vi "FAIR_GROUNDS_TEST_basaeline.vi"(1 "FIRE":bool, 2 "REVERSE":bool, 3 "Intake Motor":bool, 4 "OVERRIDE":bool, 5 "OVERRIDE 2":bool, 8 "BB1":bool, 9 "1":bool, 10 "BB2":bool, 11 "2":bool, 12 "BB3":bool, 13 "3":bool, 14 "BB4":bool) -> (20 "Ball Count":dbl, 21 "Intake motor":dbl, 22 "Motor A 2":dbl, 23 "Motor B 3":dbl, 24 "Motor C":dbl)   [LabVIEW 2011]
panel:
  in  "Prime":dbl(knob)=0.20200759564815568 scale=0.0..1.0
  in  "FIRE":dbl(knob)=0.5049245430258039 scale=0.0..1.0
  out "C from 3":bool
  out "B from 2":bool
  out "A from 1":bool
  out "BSB State":enum16{"Ball Entered"}(ring)
  out "BSC":bool
  out "BSB":bool
  out "BSA":bool
  out "MC":enum16{"Stopped", "Foward", "Reverse"}(ring)
  out "MA":enum16{"Stopped", "Foward", "Reverse"}(ring)
  out "MB":enum16{"Stopped", "Foward", "Reverse"}(ring)
  out "Intake motor":bool
  out "C Status":string
  out "B Status":string
  out "A Status":string
  out "Ball System State":string
  out "Primed":bool
  out "MA":bool
  out "MB":bool
  out "MC":bool
  # "Upper System"
  # "Upper/Middle System (U/M)"
  # "Ball systems"
  # "Vacant = Black (T)\nOccupied = Orange (F)"
  # "Lower/Middle System (L/M)"
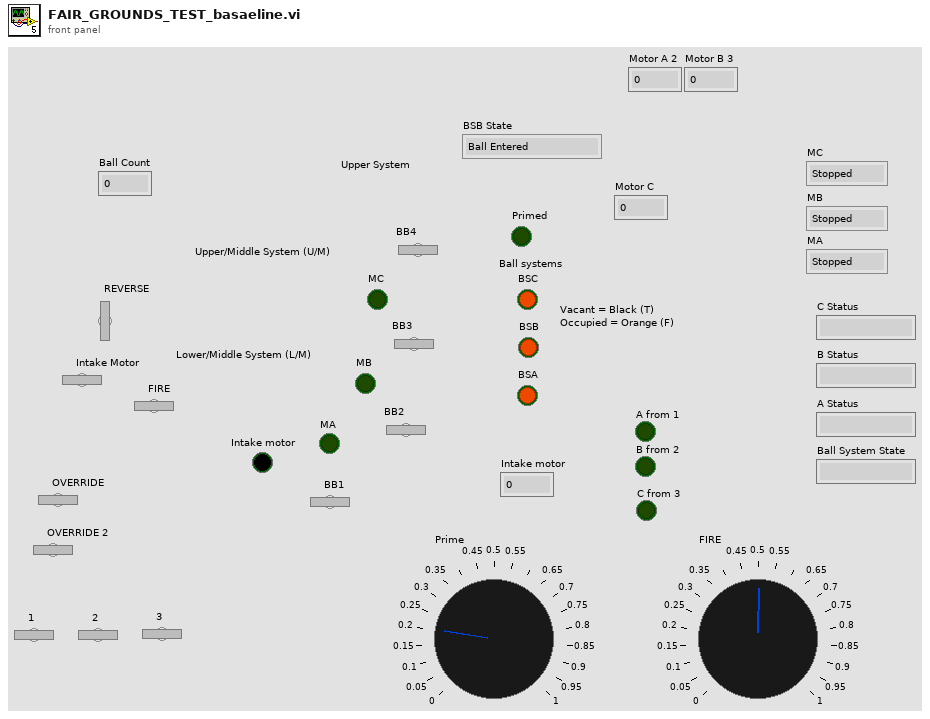
[diagram p1: front panel]
types:
  T1 = enum16{"Ball Entered", "Ball Stopped", "Ball Moveing", "Ball Leaving"}
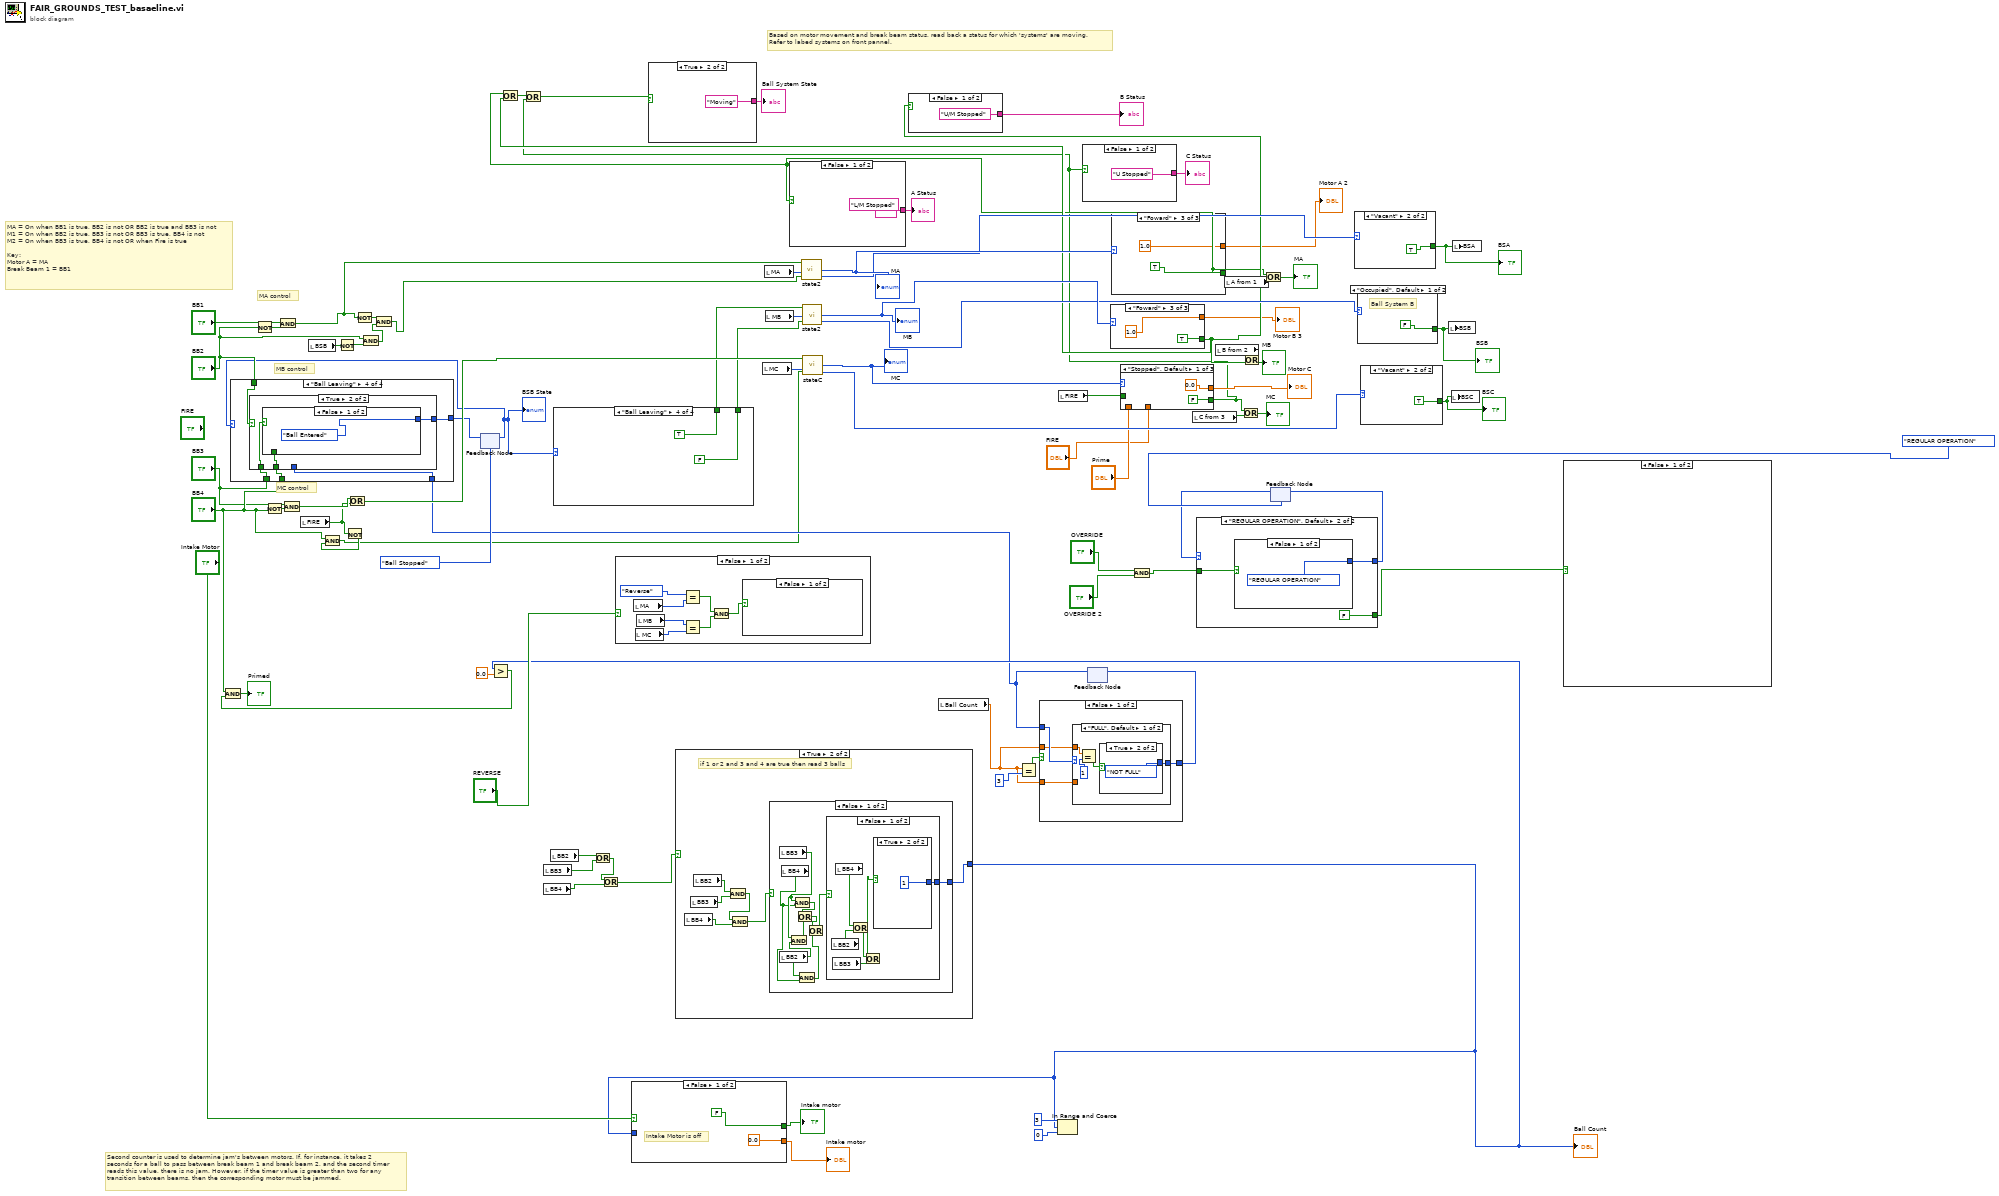
[diagram p0: block diagram]
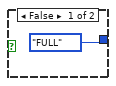
[diagram p2: hidden frame]
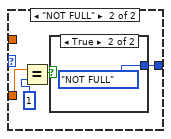
[diagram p3: hidden frame]
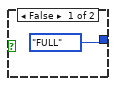
[diagram p4: hidden frame]
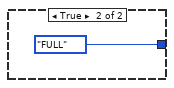
[diagram p5: hidden frame]
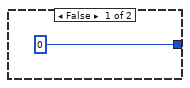
[diagram p6: hidden frame]
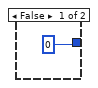
[diagram p7: hidden frame]
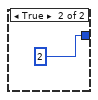
[diagram p8: hidden frame]
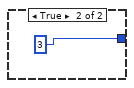
[diagram p9: hidden frame]
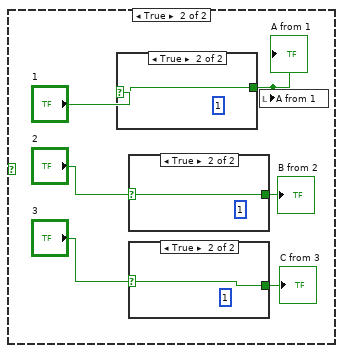
[diagram p10: hidden frame]
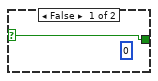
[diagram p11: hidden frame]
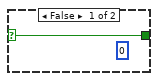
[diagram p12: hidden frame]
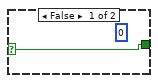
[diagram p13: hidden frame]
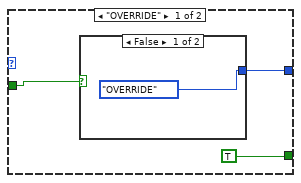
[diagram p14: hidden frame]
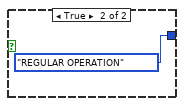
[diagram p15: hidden frame]
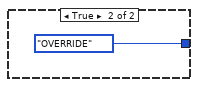
[diagram p16: hidden frame]
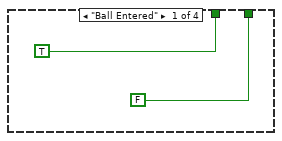
[diagram p17: hidden frame]
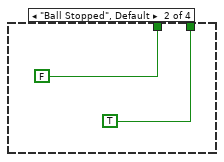
[diagram p18: hidden frame]
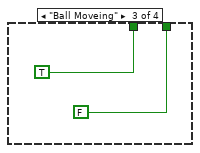
[diagram p19: hidden frame]
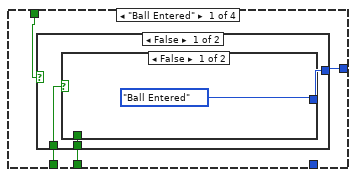
[diagram p20: hidden frame]
diagram:
  # "MC control"
  # "MB control"
  # "MA control"
  # "Second counter is used to determine jam's between motors. If, for instance, it takes 2\nseconds for a ball to pass between break beam 1 and break beam 2, and the second timer\nreads this value, there is no jam. However, if the timer value is greater than two for any\ntransition between beams, then the corresponding motor must be jammed."
  # "Based on motor movement and break beam status, read back a status for which 'systems' are moving.\nRefer to labed systems on front pannel."
  # "MA = On when BB1 is true, BB2 is not OR BB2 is true and BB3 is not\nM1 = On when BB2 is true, BB3 is not OR BB3 is true, BB4 is not\nM2 = On when BB3 is true, BB4 is not OR when Fire is true\n\nKey:\nMotor A = MA\nBreak Beam 1 = BB1"
  n1 = Not(x="BB2") -> (.not. x?=w59:bool)
  n2 = Not(x="BB4") -> (.not. x?=w58:bool)
  n3 = And(x="BB1", y=w59) -> (x .and. y?=w46:bool)
  n4 = And(x="BB3", y=w58) -> (x .and. y?=w57:bool)
  n5 = local read "FIRE"() -> (w16:bool)
  n6 = local read "BSB"() -> (w56:bool)
  n7 = Not(x=w56) -> (.not. x?=w55:bool)
  n8 = Not(x=w16) -> (.not. x?=w4:bool)
  n9 = And(x="BB4", y=w4) -> (x .and. y?=w3:bool)
  n10 = Or(x=w57, y=w16) -> (x .or. y?=w47:bool)
  n11 = Not(x=w46) -> (.not. x?=w52:bool)
  n12 = And(x="BB2", y=w55) -> (x .and. y?=w54:bool)
  n13 = And(x=w52, y=w54) -> (x .and. y?=w53:bool)
  n14 = feedback #1(T1."Ball Stopped") -> (w37:T1)
  "BSB State" <- w37
  n15 = local read "BB4"() -> (w19:bool)
  n16 = local read "BB3"() -> (w18:bool)
  n17 = local read "BB2"() -> (w20:bool)
  n18 = case shown="\"Ball Leaving\"" w37 {
    tunnel: [TRUE FALSE TRUE TRUE] -> w40
    tunnel: [FALSE TRUE FALSE FALSE] -> w39
    frame "Ball Entered" {
    }
    frame "Ball Stopped", Default {
    }
    frame "Ball Moveing" {
    }
    frame "Ball Leaving" {
    }
  }
  n19 = Or(x=w20, y=w18) -> (x .or. y?=w21:bool)
  n20 = Or(x=w21, y=w19) -> (x .or. y?=w17:bool)
  n21 = case shown="False" "REVERSE" {
    frame False {
      n22 = local read "MA"() -> (w96:enum16{"Stopped", "Foward", "Reverse"})
      n23 = local read "MC"() -> (w94:enum16{"Stopped", "Foward", "Reverse"})
      n24 = local read "MB"() -> (w95:enum16{"Stopped", "Foward", "Reverse"})
      n25 = Equal?(x=enum16{"Stopped", "Foward", "Reverse"}."Reverse" ("value"), y=w96) -> (x = y?=w92:bool)
      n26 = Equal?(x=w95, y=w94) -> (x = y?=w93:bool)
      n27 = And(x=w92, y=w93) -> (x .and. y?=w91:bool)
      n28 = case shown="False" w91 {
        frame False {
        }
        frame True {
          w98 = enum16{"Stopped", "Foward", "Reverse"}."Stopped" ("value")
          n29 = local write "MA"(w98) -> ()
          n30 = local write "MB"(w98) -> ()
          n31 = local write "MC"(w98) -> ()
        }
      }
    }
    frame True {
      w99 = enum16{"Stopped", "Foward", "Reverse"}."Reverse" ("MB")
      n32 = local write "MC"(w99) -> ()
      n33 = local write "MA"(w99) -> ()
      n34 = local write "MB"(w99) -> ()
    }
  }
  n35 = case shown="True" w17 {
    tunnel: [0 w102] -> w15
    frame False {
    }
    frame True {
      # "if 1 or 2 and 3 and 4 are true then read 3 balls"
      n36 = local read "BB4"() -> (w103:bool)
      n37 = local read "BB3"() -> (w104:bool)
      n38 = local read "BB2"() -> (w105:bool)
      n39 = And(x=w105, y=w104) -> (x .and. y?=w106:bool)
      n40 = And(x=w106, y=w103) -> (x .and. y?=w101:bool)
      n41 = case shown="False" w101 {
        tunnel: [w115 3] -> w102
        frame False {
          n42 = local read "BB3"() -> (w112:bool)
          n43 = local read "BB2"() -> (w111:bool)
          n44 = local read "BB4"() -> (w110:bool)
          n45 = And(x=w112, y=w111) -> (x .and. y?=w113:bool)
          n46 = And(x=w112, y=w110) -> (x .and. y?=w114:bool)
          n47 = Or(x=w114, y=w113) -> (x .or. y?=w109:bool)
          n48 = And(x=w111, y=w110) -> (x .and. y?=w107:bool)
          n49 = Or(x=w109, y=w107) -> (x .or. y?=w108:bool)
          n50 = case shown="False" w108 {
            tunnel: [w121 2] -> w115
            frame False {
              n51 = local read "BB2"() -> (w120:bool)
              n52 = local read "BB3"() -> (w118:bool)
              n53 = local read "BB4"() -> (w116:bool)
              n54 = Or(x=w116, y=w120) -> (x .or. y?=w119:bool)
              n55 = Or(x=w119, y=w118) -> (x .or. y?=w117:bool)
              n56 = case shown="True" w117 {
                tunnel: [0 1] -> w121
                frame False {
                }
                frame True {
                }
              }
            }
            frame True {
            }
          }
        }
        frame True {
        }
      }
    }
  }
  "Ball Count" <- w15
  n57 = Greater?(x=w15, y=0.0 ("f")) -> (0:w74:bool)
  n58 = And(x="BB4", y=w74) -> (x .and. y?=→"Primed":bool)
  n59 = case shown="False" "Intake Motor" {
    tunnel: [FALSE w130] -> w77
    tunnel: [0.0 w129] -> w50
    tunnel: w15 -> [_ w128]
    frame False {
      # "Intake Motor is off"
    }
    frame True {
      # "Only allow the intake\nmotor to be on if\nthere are less than\n3 Ballz"
      n60 = Less?(x=w128, y=3) -> (x < y?=w131:bool)
      n61 = case shown="False" w131 {
        selector: w131 -> [_ w136]
        tunnel: [TRUE w136] -> w130
        tunnel: [-1 1] -> w129
        frame False {
        }
        frame True {
        }
      }
    }
  }
  "Intake motor" <- w77
  "Intake motor" <- w50
  n62 = local read "MC"() -> (w70:enum16{"Stopped", "Foward", "Reverse"})
  n63 = local read "MA"() -> (w71:enum16{"Stopped", "Foward", "Reverse"})
  n64 = local read "MB"() -> (w72:enum16{"Stopped", "Foward", "Reverse"})
  n65 = call "state2.vi"("Stop/Transfer"=w53, "State"=w71, "Start"=w46) -> ("Ball State"=w63:enum16{"Occupied", "Vacant"}, "OutState"=w69:enum16{"Stopped", "Foward", "Reverse"})  [unwired: 1 in]
  "MA" <- w69
  n66 = call "state2.vi"("Stop/Transfer"=w39, "State"=w72, "Start"=w40) -> ("Ball State"=w64:enum16{"Occupied", "Vacant"}, "OutState"=w68:enum16{"Stopped", "Foward", "Reverse"})  [unwired: 1 in]
  "MB" <- w68
  n67 = call "stateC.vi"("Stop/Transfer"=w3, "State"=w70, "Start"=w47) -> ("Ball State"=w65:enum16{"Occupied", "Vacant"}, "OutState"=w67:enum16{"Stopped", "Foward", "Reverse"})  [unwired: 1 in]
  "MC" <- w67
  n68 = local read "Ball Count"() -> (w10:dbl)
  n69 = Equal?(x=w10, y=3) -> (x = y?=w13:bool)
  n70 = In Range and Coerce(upper limit=3, x=w15, lower limit=0) -> ()  [unwired: 2 out]
  n71 = local read "FIRE"() -> (w8:bool)
  n72 = feedback #2() -> (w11:enum16{"FULL", "NOT FULL"})  [unwired: 1 in]
  n73 = case shown="\"Ball Leaving\"" w37 {
    tunnel: "BB2" -> [w140 w160 w180 w203]
    tunnel: "BB3" -> [w139 w159 w179 w205]
    tunnel: "BB4" -> [w138 w158 w178 w204]
    tunnel: [w137 w157 w181 w206] -> w38
    tunnel: w11 -> [_ _ w177 w202]
    frame "Ball Entered" {
      n74 = case shown="False" w140 {
        tunnel: [w143 w151] -> w137
        tunnel: w139 -> [w142 w149]
        tunnel: w138 -> [w141 w150]
        frame False {
          n75 = case shown="False" w142 {
            tunnel: [T1."Ball Entered" w146] -> w143
            tunnel: w141 -> [_ w145]
            frame False {
            }
            frame True {
              n76 = case shown="False" w145 {
                tunnel: [T1."Ball Leaving" T1."Ball Stopped"] -> w146
                frame False {
                }
                frame True {
                }
              }
            }
          }
        }
        frame True {
          n77 = case shown="False" w149 {
            tunnel: [T1."Ball Entered" w154] -> w151
            tunnel: w150 -> [_ w153]
            frame False {
            }
            frame True {
              n78 = case shown="False" w153 {
                tunnel: [T1."Ball Leaving" T1."Ball Stopped"] -> w154
                frame False {
                }
                frame True {
                }
              }
            }
          }
        }
      }
    }
    frame "Ball Stopped", Default {
      n79 = case shown="True" w160 {
        tunnel: [w163 w171] -> w157
        tunnel: w159 -> [w162 w169]
        tunnel: w158 -> [w161 w170]
        frame False {
          n80 = case shown="False" w162 {
            tunnel: [T1."Ball Stopped" w166] -> w163
            tunnel: w161 -> [_ w165]
            frame False {
            }
            frame True {
              n81 = case shown="True" w165 {
                tunnel: [T1."Ball Leaving" T1."Ball Stopped"] -> w166
                frame False {
                }
                frame True {
                }
              }
            }
          }
        }
        frame True {
          n82 = case shown="False" w169 {
            tunnel: [T1."Ball Entered" w174] -> w171
            tunnel: w170 -> [_ w173]
            frame False {
            }
            frame True {
              n83 = case shown="True" w173 {
                tunnel: [T1."Ball Leaving" T1."Ball Stopped"] -> w174
                frame False {
                }
                frame True {
                }
              }
            }
          }
        }
      }
    }
    frame "Ball Moveing" {
      n84 = case shown="False" w180 {
        tunnel: [w185 w196] -> w181
        tunnel: w179 -> [w184 w194]
        tunnel: w178 -> [w183 w195]
        tunnel: w177 -> [w182 _]
        frame False {
          n85 = case shown="False" w184 {
            tunnel: [w187 w191] -> w185
            tunnel: w183 -> [_ w190]
            tunnel: w182 -> [w186 _]
            frame False {
              n86 = case shown="\"NOT FULL\"" w186 {
                tunnel: [T1."Ball Moveing" T1."Ball Stopped"] -> w187
                frame "FULL", Default {
                }
                frame "NOT FULL" {
                }
              }
            }
            frame True {
              n87 = case shown="True" w190 {
                tunnel: [T1."Ball Moveing" T1."Ball Stopped"] -> w191
                frame False {
                }
                frame True {
                }
              }
            }
          }
        }
        frame True {
          n88 = case shown="False" w194 {
            tunnel: [T1."Ball Entered" w199] -> w196
            tunnel: w195 -> [_ w198]
            frame False {
            }
            frame True {
              n89 = case shown="False" w198 {
                tunnel: [T1."Ball Leaving" T1."Ball Stopped"] -> w199
                frame False {
                }
                frame True {
                }
              }
            }
          }
        }
      }
    }
    frame "Ball Leaving" {
      n90 = case shown="True" w203 {
        tunnel: [w210 w221] -> w206
        tunnel: w205 -> [w209 w219]
        tunnel: w204 -> [w208 w220]
        tunnel: w202 -> [w207 _]
        frame False {
          n91 = case shown="False" w209 {
            tunnel: [w212 w216] -> w210
            tunnel: w208 -> [_ w215]
            tunnel: w207 -> [w211 _]
            frame False {
              n92 = case shown="\"NOT FULL\"" w211 {
                tunnel: [T1."Ball Moveing" T1."Ball Stopped"] -> w212
                frame "FULL", Default {
                }
                frame "NOT FULL" {
                }
              }
            }
            frame True {
              n93 = case shown="True" w215 {
                tunnel: [T1."Ball Leaving" T1."Ball Stopped"] -> w216
                frame False {
                }
                frame True {
                }
              }
            }
          }
        }
        frame True {
          n94 = case shown="False" w219 {
            tunnel: [T1."Ball Entered" w224] -> w221
            tunnel: w220 -> [_ w223]
            frame False {
            }
            frame True {
              n95 = case shown="False" w223 {
                tunnel: [T1."Ball Leaving" T1."Ball Stopped"] -> w224
                frame False {
                }
                frame True {
                }
              }
            }
          }
        }
      }
    }
  }
  n96 = feedback-in #1(w38) -> ()
  n97 = case shown="False" w13 {
    tunnel: w11 -> [w230 _]
    tunnel: [w229 enum16{"FULL", "NOT FULL"}."FULL"] -> w12
    tunnel: w10 -> [w228 _]
    tunnel: w10 -> [w227 _]
    frame False {
      n98 = case shown="\"FULL\", Default" w230 {
        tunnel: [w231 w240] -> w229
        tunnel: w228 -> [_ w239]
        tunnel: w227 -> [w232 _]
        frame "FULL", Default {
          n99 = Equal?(x=w232, y=1) -> (x = y?=w234:bool)
          n100 = case shown="True" w234 {
            tunnel: [enum16{"FULL", "NOT FULL"}."FULL" enum16{"FULL", "NOT FULL"}."NOT FULL"] -> w231
            frame False {
            }
            frame True {
            }
          }
        }
        frame "NOT FULL" {
          n101 = Equal?(x=w239, y=1) -> (x = y?=w238:bool)
          n102 = case shown="True" w238 {
            tunnel: [enum16{"FULL", "NOT FULL"}."FULL" enum16{"FULL", "NOT FULL"}."NOT FULL"] -> w240
            frame False {
            }
            frame True {
            }
          }
        }
      }
    }
    frame True {
    }
  }
  n103 = feedback-in #2(w12) -> ()
  n104 = case shown="\"Foward\"" w68 {
    tunnel: [FALSE TRUE TRUE] -> w45
    tunnel: [0.0 -1.0 1.0] -> w1
    frame "Stopped", Default {
    }
    frame "Reverse" {
    }
    frame "Foward" {
    }
  }
  "Motor B 3" <- w1
  n105 = case shown="False" w45 {
    tunnel: ["U/M Stopped" "U/M Moving"] -> w79
    frame False {
    }
    frame True {
    }
  }
  "B Status" <- w79
  n106 = case shown="\"Foward\"" w69 {
    tunnel: [FALSE TRUE TRUE] -> w35
    tunnel: [0.0 -1.0 1.0] -> w2
    frame "Stopped", Default {
    }
    frame "Reverse" {
    }
    frame "Foward" {
    }
  }
  "Motor A 2" <- w2
  n107 = Or(x=w35, y=w45) -> (x .or. y?=w49:bool)
  n108 = case shown="False" w35 {
    tunnel: ["L/M Stopped" "L/M Moving up"] -> w80
    frame False {
    }
    frame True {
    }
  }
  "A Status" <- w80
  n109 = case shown="\"Stopped\", Default" w67 {
    tunnel: [0.0 w264 -1.0] -> w66
    tunnel: [FALSE TRUE TRUE] -> w29
    tunnel: "Prime" -> [_ w262 _]
    tunnel: w8 -> [_ w265 _]
    tunnel: "FIRE" -> [_ w263 _]
    frame "Stopped", Default {
    }
    frame "Foward" {
      n110 = case shown="False" w265 {
        tunnel: [w267 w268] -> w264
        tunnel: w263 -> [_ w268]
        tunnel: w262 -> [w267 _]
        frame False {
        }
        frame True {
        }
      }
    }
    frame "Reverse" {
    }
  }
  "Motor C" <- w66
  n111 = Or(x=w49, y=w29) -> (x .or. y?=w48:bool)
  n112 = case shown="True" w48 {
    tunnel: ["Stopped" "Moving"] -> w81
    frame False {
    }
    frame True {
    }
  }
  "Ball System State" <- w81
  n113 = case shown="False" w29 {
    tunnel: ["U Stopped" "Firing"] -> w78
    frame False {
    }
    frame True {
    }
  }
  "C Status" <- w78
  n114 = And(x="OVERRIDE", y="OVERRIDE 2") -> (x .and. y?=w25:bool)
  n115 = local read "C from 3"() -> (w28:bool)
  n116 = local read "B from 2"() -> (w31:bool)
  n117 = local read "A from 1"() -> (w32:bool)
  n118 = Or(x=w29, y=w28) -> (x .or. y?=→"MC":bool)
  n119 = Or(x=w31, y=w45) -> (x .or. y?=→"MB":bool)
  n120 = Or(x=w35, y=w32) -> (x .or. y?=→"MA":bool)
  n121 = feedback #3(enum16{"OVERRIDE", "REGULAR OPERATION"}."REGULAR OPERATION") -> (w26:enum16{"OVERRIDE", "REGULAR OPERATION"})
  n122 = case shown="\"REGULAR OPERATION\", Default" w26 {
    tunnel: [w276 w282] -> w27
    tunnel: w25 -> [w277 w281]
    tunnel: [TRUE FALSE] -> w24
    frame "OVERRIDE" {
      n123 = case shown="False" w277 {
        tunnel: [enum16{"OVERRIDE", "REGULAR OPERATION"}."OVERRIDE" enum16{"OVERRIDE", "REGULAR OPERATION"}."REGULAR OPERATION"] -> w276
        frame False {
        }
        frame True {
        }
      }
    }
    frame "REGULAR OPERATION", Default {
      n124 = case shown="False" w281 {
        tunnel: [enum16{"OVERRIDE", "REGULAR OPERATION"}."REGULAR OPERATION" enum16{"OVERRIDE", "REGULAR OPERATION"}."OVERRIDE"] -> w282
        frame False {
        }
        frame True {
        }
      }
    }
  }
  n125 = feedback-in #3(w27) -> ()
  n126 = case shown="\"Vacant\"" w63 {
    tunnel: [FALSE TRUE] -> w61
    frame "Occupied", Default {
      # "Ball System A"
    }
    frame "Vacant" {
    }
  }
  "BSA" <- w61
  n127 = case shown="\"Occupied\", Default" w64 {
    tunnel: [FALSE TRUE] -> w62
    frame "Occupied", Default {
      # "Ball System B"
    }
    frame "Vacant" {
    }
  }
  "BSB" <- w62
  n128 = case shown="\"Vacant\"" w65 {
    tunnel: [FALSE TRUE] -> w60
    frame "Occupied", Default {
      # "Ball System C"
    }
    frame "Vacant" {
    }
  }
  "BSC" <- w60
  n129 = local write "BSB"(w62) -> ()
  n130 = local write "BSC"(w60) -> ()
  n131 = local write "BSA"(w61) -> ()
  n132 = case shown="False" w24 {
    frame False {
    }
    frame True {
      n133 = case shown="True" "1" {
        selector: "1" -> [w301 w302]
        tunnel: [w301 w302] -> w293
        frame False {
          (unwired) 0
        }
        frame True {
          (unwired) 1
        }
      }
      "A from 1" <- w293
      n134 = case shown="True" "2" {
        selector: "2" -> [w299 w300]
        tunnel: [w299 w300] -> w291
        frame False {
          (unwired) 0
        }
        frame True {
          (unwired) 1
        }
      }
      "B from 2" <- w291
      n135 = case shown="True" "3" {
        selector: "3" -> [w297 w298]
        tunnel: [w297 w298] -> w292
        frame False {
          (unwired) 0
        }
        frame True {
          (unwired) 1
        }
      }
      "C from 3" <- w292
      n136 = local write "A from 1"(w293) -> ()
    }
  }
